vi "dds_host_denzal-final.vi"() -> ()   [LabVIEW 2018]
uses:
  <vilib>/FPGAPlugInAG/PCIe-7841R/niLvFpga_Open_PCIe-7841R.vi
  <vilib>/rvi/interface/common/dynamic/niFpgaDynamicAddResources.vi
  <vilib>/FPGAPlugInAG/Dynamic/niLvFpga_Run_Dynamic.vi
  <vilib>/Utility/error.llb/Error Cluster From Error Code.vi
  <vilib>/rvi/errors/niLvFpgaAdjustHostInterfaceError.vi
  <vilib>/FPGAPlugInAG/Dynamic/niLvFpga_Close_Dynamic.vi
  <vilib>/rvi/interface/nirviOpenFPGA/nirviOpenFPGA.xnode
  FPGA Bitfiles/dds_FPGATarget_ddsfpga_kTR-VUpZgFc _denzal-final.lvbitx
  <vilib>/rvi/interface/nirviMethod/nirviMethod.xnode
  <vilib>/rvi/interface/nirviReadWriteControl/nirviReadWriteControl.xnode
  <vilib>/rvi/interface/nirviCloseFPGA/nirviCloseFPGA.xnode
  <vilib>/rvi/interface/Simulation/niFpgaSimulationCallBeginRW.vi
  NiFpgaLv.dll
  <vilib>/rvi/Analysis/host/Public/NI_FpgaMspHost.lvlib
panel:
  in  "set xz drive":bool
  in  "set yz drive":bool
  out "phi_dc_offset 2":fxp<+/-,17,9>
  out "Actual loop rate 2":u32
  out "Actual Sample Rate (S/s) 2":dbl=952380.9523809524 format="%#_6p"
  in  "change_phi_offset":bool
  in  "filter":bool
  in  "RMS":u16
  in  "noise_scale":fxp<+/-,16,1>
  in  "noise":bool
  out "sine_gen":dbl(graph)
  out "In Range?":bool
  in  "reset_accum":bool
  in  "frequency":u32=100
  in  "sine_amp":dbl=10.0 format="%#_13g"
  in  "xy_amplitude_mod?":bool
  in  "subtract_cross_pol_phi_mean":bool
  in  "phi_fb_out_scale":dbl
  in  "change_phi_dg":bool
  in  "phi_pg":fxp<+/-,16,12>
  in  "change_pm_freq":bool
  in  "phi_dc_offset":fxp<+/-,16,8>
  in  "test_phase_mod":bool
  in  "inst_freq_offset":fxp<+/-,33,18>
  in  "phi_lower_lim":fxp<+/-,16,16>=-1.0
  in  "phi_upper_lim":fxp<+/-,16,16>=1.0
  in  "phi_dg":dbl
  out "phi_fb_out":dbl(graph)
  out "inst_freq":dbl(graph)=22820.240234375
  in  "phi_bitshift":i16
  in  "initialize_phase_mod":bool
  in  "phase_mod":bool
  in  "phase_mod_scale":dbl
  out "phase_out":dbl(graph)=22820.240234375
  in  "phase_mod_param":T1={"Sine wave frequency (Hz)"=50.0, "Phase offset (deg)"=0.0} {"Phase offset (deg)" format="%#_6p"; "Sine wave frequency (Hz)" format="%#_6p"}
  in  "downsample_num":i16=1
  out "cross_pol_phi":dbl(graph)=22820.240234375
  out "actual_analog_in_loop_time":u32=4
  in  "desired_AI_loop_time(uSec)":u32=5
  in  "reset_phi":bool
  in  "discont_pos":fxp<+/-,17,3>=1.0
  in  "discont_neg":fxp<+/-,64,32>=-1.0
  in  "counter_offset":u8
  out "cross_pol_amp":i16(graph)=1
  in  "subtract_mean?":bool=TRUE
  out "slow_freq":dbl=50.0
  out "scale factor_slow-dds":fxp<+/-,16,1>
  in  "vpp_slow-dds":dbl
  in  "slow-dds_param":T1={"Sine wave frequency (Hz)"=50.0, "Phase offset (deg)"=0.0} {"Phase offset (deg)" format="%#_6p"; "Sine wave frequency (Hz)" format="%#_6p"}
  in  "z_slow-dds?":bool
  in  "45_sin":bool=TRUE
  in  "23_sin":bool
  in  "01_sin":bool=TRUE
  in  "just x?":bool
  out "synth_settings_client":dbl[](array[numeric])=[8.0, 50000.0]
  out "scale factor 45":fxp<+/-,16,1>
  out "scale factor 23":fxp<+/-,16,1>
  out "scale factor 01":fxp<+/-,16,1>
  in  "set xy drive":bool
  in  "vpp 45":dbl
  in  "vpp 23":dbl
  in  "vpp 01":dbl
  in  "Desired loop rate (ticks)":u32=88
  in  "frequency increment":dbl=1.0
  out "requested_freq":dbl(graph)=4000.0
  out "Sampling Rate\nAchieved?":bool=TRUE
  out "Actual Sample Rate (S/s)":dbl=952380.9523809524 format="%#_6p"
  in  "re-initialize_dds":bool
  in  "fast-dds_param":T1={"Sine wave frequency (Hz)"=4000.0, "Phase offset (deg)"=0.0} {"Phase offset (deg)" format="%#_6p"; "Sine wave frequency (Hz)" format="%#_6p"}
  in  "step_time (ms)":u32=1
  out "error out":errorcluster={"status"=FALSE, "code"=61003, "source"="niLvFpga_Run_Dynamic.vi"}
  in  "stop":bool
  # "SINE"
  # "COSINE"
  # "SINE"
types:
  T1 = cluster{"Sine wave frequency (Hz)":dbl, "Phase offset (deg)":dbl}
  T2 = enum16{"open", "replace", "create", "open or create", "replace or create", "replace or create with confirmation"}
  T3 = cluster{"frequency (periods/tick)":fxp<+,32,0>, "phase offset (periods)":fxp<+,32,0>, fxp<+/-,16,1>, fxp<+,1,1>}
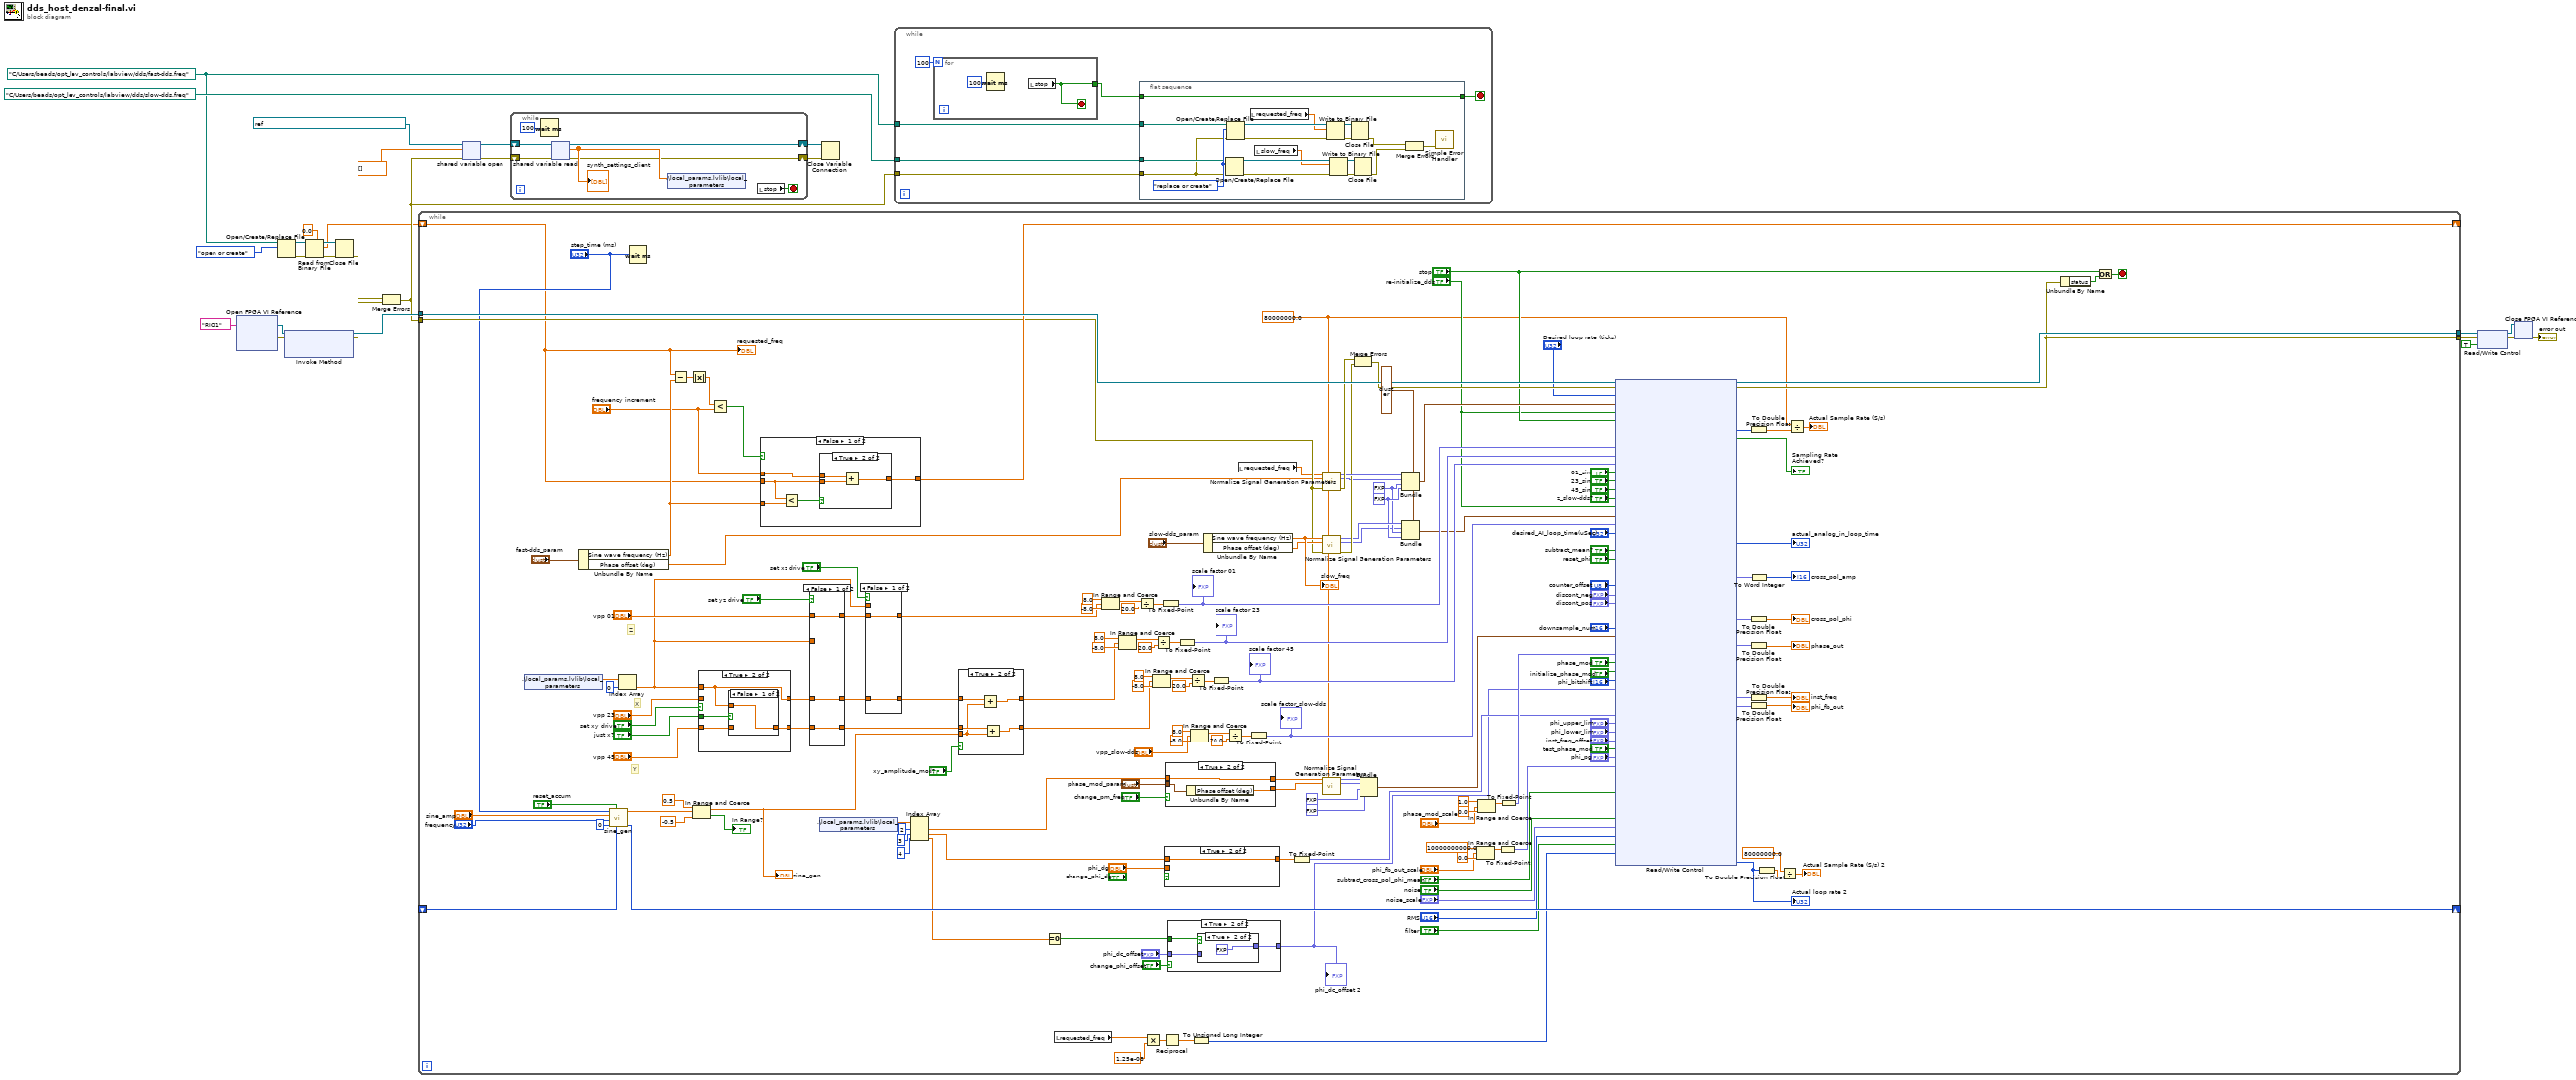
[diagram p0: block diagram]
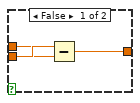
[diagram p8: hidden frame]
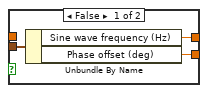
[diagram p10: hidden frame]
diagram:
  w11 = path "C:/Users/beads/opt_lev_controls/labview/dds/fast-dds.freq" ("file path (use dialog)")
  n1 = xnode "Open FPGA VI Reference"("resource name"=tag "RIO1") -> ("FPGA VI Reference Out"=w26:refnum<k20>, "error out"=w27:errorcluster)  [unwired: 1 in]
  n2 = Open/Create/Replace File(file path (use dialog)=w11, operation (0:open)=T2."open or create") -> (refnum out=w9:refnum<file>, error out=w10:errorcluster)  [unwired: 4 in, 1 out]
  n3 = xnode "Invoke Method"("FPGA VI Reference In"=w26, "error in"=w27) -> ("FPGA VI Reference Out"=w25:refnum<k20>, "error out"=w6:errorcluster)  [unwired: 1 in]
  n4 = Read from Binary File(5:0.0, 8:w10, 11:w9) -> (0:w8:errorcluster, 2:w1:dbl, 3:w7:refnum<file>)  [unwired: 3 in, 1 out]
  n5 = Close File(refnum=w7, error in=w8) -> (error out=w5:errorcluster)  [unwired: 1 out]
  n6 = Merge Errors(w5, w6) -> (w2:errorcluster)
  n7 = while {
    tunnel: w25 -> [w202]
    tunnel: w2 -> [w155]
    tunnel: [w200] -> w24
    tunnel: [w201] -> w23
    shift-right: [w180] -> _
    shift-left: w1 -> [w46]
    shift-right: [w67] -> _
    shift-left: _ -> [w66]
    stop <- w198 stop-if-true
    w150 = fxp<+/-,16,1> 0.0
    w153 = T3 {"frequency (periods/tick)"=0.0, "phase offset (periods)"=0.0, 0.0, 0.0} ("cluster")
    w151 = fxp<+,1,1> 0.0
    w121 = 80000000.0 ("FPGA clock rate (Hz)")
    # "Y"
    # "X"
    # "Z"
    n8 = shared-variable ".\\local_params.lvlib\\local_parameters"() -> (w179:dbl[])  [unwired: 1 in, 1 out]
    n9 = Unbundle By Name("fast-dds_param") -> ("Sine wave frequency (Hz)"=w184:dbl, "Phase offset (deg)"=w127:dbl)
    n10 = call "sine_gen.vi"("prev_val"=w66, "reset_accum"="reset_accum", "phase_shift 2"=u32 0, "frequency"="frequency", "sine_amp"="sine_amp", "step_time(ms)"="step_time (ms)") -> ("next_val"=w67:u32, "sine_out"=w61:dbl)  [unwired: 3 in]
    n11 = Index Array(array=w179, index=0) -> (element=w36:dbl)
    n12 = Wait (ms)(milliseconds to wait="step_time (ms)") -> ()  [unwired: 1 out]
    n13 = Subtract(x=w46, y=w184) -> (x-y=w95:dbl)
    n14 = Absolute Value(x=w95) -> (abs(x)=w94:dbl)
    n15 = In Range and Coerce(upper limit=0.5, x=w61, lower limit=-0.5) -> (coerced(x)=w62:dbl, In Range?=→"In Range?":bool)
    "sine_gen" <- w62
    n16 = case shown="True" "set xy drive" {
      tunnel: "vpp 23" -> [w245 _]
      tunnel: [w245 w246] -> w39
      tunnel: "vpp 45" -> [w244 w248]
      tunnel: [w244 w247] -> w38
      tunnel: "just x?" -> [_ w249]
      tunnel: w36 -> [_ w246]
      frame False {
      }
      frame True {
        n17 = case shown="False" w249 {
          tunnel: w248 -> [_ w251]
          tunnel: [w250 w251] -> w247
          tunnel: w246 -> [w250 _]
          frame False {
          }
          frame True {
          }
        }
      }
    }
    n18 = Less?(x=w94, y="frequency increment") -> (x < y?=w92:bool)
    n19 = case shown="False" w92 {
      tunnel: [w227 w237] -> w180
      tunnel: w46 -> [w226 _]
      tunnel: w184 -> [w230 w237]
      tunnel: "frequency increment" -> [w228 _]
      frame False {
        n20 = Less?(x=w226, y=w230) -> (x < y?=w229:bool)
        n21 = case shown="True" w229 {
          tunnel: w226 -> [w232 w236]
          tunnel: w228 -> [w231 w235]
          tunnel: [w233 w234] -> w227
          frame False {
            n22 = Subtract(x=w232, y=w231) -> (x-y=w233:dbl)
          }
          frame True {
            n23 = Add(x=w235, y=w236) -> (x+y=w234:dbl)
          }
        }
      }
      frame True {
      }
    }
    n24 = case shown="False" "set yz drive" {
      tunnel: [w208 w210] -> w35
      tunnel: "vpp 01" -> [w208 _]
      tunnel: w36 -> [_ w210]
      tunnel: [w207 w209] -> w32
      tunnel: w39 -> [w207 w209]
      tunnel: [w206 w210] -> w31
      tunnel: w38 -> [w206 _]
      frame False {
      }
      frame True {
      }
    }
    n25 = shared-variable ".\\local_params.lvlib\\local_parameters"() -> (w99:dbl[])  [unwired: 1 in, 1 out]
    n26 = case shown="False" "set xz drive" {
      tunnel: w36 -> [_ w205]
      tunnel: w35 -> [w204 _]
      tunnel: [w204 w205] -> w34
      tunnel: [w203 w205] -> w33
      tunnel: w32 -> [w203 _]
      frame False {
      }
      frame True {
      }
    }
    n27 = Index Array(array=w99, index #1=2 ("index"), index #2=3 ("index"), index #3=4 ("index")) -> (element #1=w97:dbl, element #2=w89:dbl, element #3=w42:dbl)
    n28 = case shown="True" "xy_amplitude_mod?" {
      tunnel: w33 -> [w218 w223]
      tunnel: [w218 w221] -> w75
      tunnel: w31 -> [w217 w222]
      tunnel: [w217 w220] -> w74
      tunnel: w62 -> [_ w219]
      frame False {
      }
      frame True {
        n29 = Add(x=w223, y=w219) -> (x+y=w221:dbl)
        n30 = Add(x=w222, y=w219) -> (x+y=w220:dbl)
      }
    }
    n31 = Equal To 0?(x=w42) -> (x = 0?=w53:bool)
    n32 = local read "requested_freq"() -> (w29:dbl)
    n33 = In Range and Coerce(upper limit=8.0, x=w34, lower limit=-8.0) -> (coerced(x)=w187:dbl)  [unwired: 1 out]
    n34 = In Range and Coerce(upper limit=8.0, x=w75, lower limit=-8.0) -> (coerced(x)=w168:dbl)  [unwired: 1 out]
    n35 = Divide(x=w187, y=20.0) -> (x/y=w193:dbl)
    n36 = Multiply(x=w29, y=1.25e-08) -> (x*y=w45:dbl)
    n37 = In Range and Coerce(upper limit=8.0, x=w74, lower limit=-8.0) -> (coerced(x)=w162:dbl)  [unwired: 1 out]
    n38 = Divide(x=w168, y=20.0) -> (x/y=w169:dbl)
    n39 = To Fixed-Point(number=w193) -> (fixed-point=w182:fxp<+/-,16,1>)  [unwired: 1 in]
    "scale factor 01" <- w182
    n40 = Reciprocal(x=w45) -> (1/x=w44:dbl)
    n41 = case shown="True" "change_phi_dg" {
      tunnel: w89 -> [_ w225]
      tunnel: [w224 w225] -> w88
      tunnel: "phi_dg" -> [w224 _]
      frame False {
      }
      frame True {
      }
    }
    n42 = case shown="True" "change_pm_freq" {
      tunnel: "phase_mod_param" -> [w240 w243]
      tunnel: [w239 w242] -> w123
      tunnel: [w238 w241] -> w122
      tunnel: w97 -> [_ w242]
      frame False {
        n43 = Unbundle By Name(w240) -> ("Sine wave frequency (Hz)"=w239:dbl, "Phase offset (deg)"=w238:dbl)
      }
      frame True {
        n44 = Unbundle By Name(w243) -> ("Phase offset (deg)"=w241:dbl)
      }
    }
    n45 = case shown="True" "change_phi_offset" {
      tunnel: [w211 w213] -> w55
      tunnel: "phi_dc_offset" -> [w211 w212]
      tunnel: w53 -> [_ w214]
      frame False {
      }
      frame True {
        n46 = case shown="True" w214 {
          tunnel: [w215 fxp<+/-,16,8> 0.0] -> w213
          tunnel: w212 -> [w215 _]
          frame False {
          }
          frame True {
          }
        }
      }
    }
    "phi_dc_offset 2" <- w55
    n47 = To Fixed-Point(number=w169) -> (fixed-point=w165:fxp<+/-,16,1>)  [unwired: 1 in]
    "scale factor 23" <- w165
    n48 = Divide(x=w162, y=20.0) -> (x/y=w163:dbl)
    n49 = In Range and Coerce(upper limit=8.0, x="vpp_slow-dds", lower limit=-8.0) -> (coerced(x)=w146:dbl)  [unwired: 1 out]
    n50 = To Unsigned Long Integer(number=w44) -> (unsigned 32bit integer=w48:u32)
    n51 = Unbundle By Name("slow-dds_param") -> ("Sine wave frequency (Hz)"=w157:dbl, "Phase offset (deg)"=w156:dbl)
    "slow_freq" <- w157
    n52 = To Fixed-Point(number=w163) -> (fixed-point=w159:fxp<+/-,16,1>)  [unwired: 1 in]
    "scale factor 45" <- w159
    n53 = Divide(x=w146, y=20.0) -> (x/y=w147:dbl)
    n54 = local read "requested_freq"() -> (w30:dbl)
    n55 = To Fixed-Point(number=w147) -> (fixed-point=w142:fxp<+/-,16,1>)  [unwired: 1 in]
    "scale factor_slow-dds" <- w142
    n56 = To Fixed-Point(number=w88) -> (fixed-point=w85:fxp<+/-,32,16>)  [unwired: 1 in]
    n57 = call <vilib>:"Normalize Signal Generation Parameters.vi"("frequency (Hz)"=w30, "FPGA clock rate (Hz)"=w121, "phase offset (deg)"=w127, "error in (no error)"=w155) -> ("frequency (periods/tick)"=w195:fxp<+,32,0>, "phase offset (periods)"=w125:fxp<+,32,0>, "error out"=w197:errorcluster)  [unwired: 6 in, 3 out]
    n58 = call <vilib>:"Normalize Signal Generation Parameters.vi"("frequency (Hz)"=w157, "FPGA clock rate (Hz)"=w121, "phase offset (deg)"=w156, "error in (no error)"=w155) -> ("frequency (periods/tick)"=w152:fxp<+,32,0>, "phase offset (periods)"=w126:fxp<+,32,0>, "error out"=w154:errorcluster)  [unwired: 6 in, 3 out]
    n59 = call <vilib>:"Normalize Signal Generation Parameters.vi"("frequency (Hz)"=w123, "FPGA clock rate (Hz)"=w121, "phase offset (deg)"=w122) -> ("frequency (periods/tick)"=w120:fxp<+,32,0>, "phase offset (periods)"=w119:fxp<+,32,0>)  [unwired: 7 in, 4 out]
    n60 = Merge Errors(w197, w154) -> (w196:errorcluster)
    n61 = Bundle("frequency (periods/tick)"=w120, "phase offset (periods)"=w119, fxp<+/-,16,1> 0.0, fxp<+,1,1> 0.0) -> (w118:T3)  [unwired: 1 in]
    n62 = Bundle(cluster=w153, "frequency (periods/tick)"=w195, "phase offset (periods)"=w125, w150, w151) -> (w192:T3)
    n63 = Bundle(cluster=w153, "frequency (periods/tick)"=w152, "phase offset (periods)"=w126, w150, w151) -> (w149:T3)
    n64 = In Range and Coerce(upper limit=10000000000.0, x="phi_fb_out_scale", lower limit=0.0) -> (coerced(x)=w81:dbl)  [unwired: 1 out]
    n65 = In Range and Coerce(upper limit=1.0, x="phase_mod_scale", lower limit=0.0) -> (coerced(x)=w111:dbl)  [unwired: 1 out]
    n66 = To Fixed-Point(number=w81) -> (fixed-point=w80:fxp<+/-,16,16>)  [unwired: 1 in]
    n67 = To Fixed-Point(number=w111) -> (fixed-point=w91:fxp<+,16,0>)  [unwired: 1 in]
    n68 = xnode "Read/Write Control"("FPGA VI Reference In"=w202, "error in"=w196, "Desired loop rate (ticks)"="Desired loop rate (ticks)", "sinewave-props_fast-dds"=w192, "Initialize fast-dds"="re-initialize_dds", "stop"="stop", "fast-dds_scale01"=w182, "fast-dds_scale23"=w165, "fast-dds_scale45"=w159, "01_sin"="01_sin", "23_sin"="23_sin", "45_sin"="45_sin", "z_slow-dds?"="z_slow-dds?", "Initialize slow-dds"="re-initialize_dds", "sinewave-props_slow-dds"=w149, "slow-dds_scale"=w142, "desired_analog_in_loop_time_(uSec)"="desired_AI_loop_time(uSec)", "subtract_mean"="subtract_mean?", "reset_phi"="reset_phi", "counter_offset"="counter_offset", "discont_neg"="discont_neg", "discont_pos"="discont_pos", "downsample_num"="downsample_num", "phase_mod_props"=w118, "phase_mod_scale"=w91, "phase_mod"="phase_mod", "initialize_phase_mod"="initialize_phase_mod", "phi_bitshift"="phi_bitshift", "phi_dc_offset"=w55, "phi_dg"=w85, "phi_upper_lim"="phi_upper_lim", "phi_lower_lim"="phi_lower_lim", "inst_freq_offset"="inst_freq_offset", "test_phase_mod"="test_phase_mod", "phi_pg"="phi_pg", "phi_fb_out_scale"=w80, "subtract_cross_pol_phi_mean"="subtract_cross_pol_phi_mean", "noise"="noise", "noise_scale"="noise_scale", "RMS"="RMS", "filter"="filter", "Desired loop rate (ticks) 2"=w48) -> ("FPGA VI Reference Out"=w201:refnum<k20>, "error out"=w200:errorcluster, "Actual loop rate"=w189:u32, "Sampling rate achieved?"=→"Sampling Rate\nAchieved?":bool, "actual_analog_in_loop_time"=→"actual_analog_in_loop_time":u32, "cross_pol_amp"=w140:fxp<+,32,16>, "phi_full_out"=w131:fxp<+/-,35,21>, "phase_mod_out"=w115:fxp<+/-,49,17>, "inst_freq"=w107:fxp<+/-,35,20>, "phi_fb_out"=w104:fxp<+/-,32,0>, "Actual loop rate 2"=w50:u32)  [unwired: 1 in, 5 out]
    "Actual loop rate 2" <- w50
    n69 = To Double Precision Float(number=w189) -> (double precision float=w191:dbl)
    n70 = To Word Integer(number=w140) -> (16bit integer=→"cross_pol_amp":i16)
    n71 = To Double Precision Float(number=w131) -> (double precision float=→"cross_pol_phi":dbl)
    n72 = To Double Precision Float(number=w115) -> (double precision float=→"phase_out":dbl)
    n73 = To Double Precision Float(number=w107) -> (double precision float=→"inst_freq":dbl)
    n74 = To Double Precision Float(number=w104) -> (double precision float=→"phi_fb_out":dbl)
    n75 = To Double Precision Float(number=w50) -> (double precision float=w52:dbl)
    n76 = Divide(x=80000000.0, y=w52) -> (x/y=→"Actual Sample Rate (S/s) 2":dbl)
    n77 = Divide(x=w121, y=w191) -> (x/y=→"Actual Sample Rate (S/s)":dbl)
    n78 = Unbundle By Name(w200) -> ("status"=w199:bool)
    n79 = Or(x="stop", y=w199) -> (x .or. y?=w198:bool)
    "requested_freq" <- w46
  }
  n80 = shared-variable-open(refnum<k21> "ni.var.psp://localhost/daq_lib/synth_settings" ("shared variable refnum in"), w2, dbl[] [] ("synth_settings_client")) -> (w16:refnum<k21>, w15:errorcluster)  [unwired: 1 in]
  n81 = while {
    shift-right: [w253] -> w14
    shift-left: w16 -> [w256]
    shift-right: [w252] -> w13
    shift-left: w15 -> [w255]
    stop <- w257 stop-if-true
    n82 = Wait (ms)(milliseconds to wait=u32 100) -> ()  [unwired: 1 out]
    n83 = shared-variable-read(w256, w255) -> (w253:refnum<k21>, w252:errorcluster, w254:dbl[])  [unwired: 1 out]
    "synth_settings_client" <- w254
    n84 = shared-variable ".\\local_params.lvlib\\local_parameters"(w254) -> ()  [unwired: 1 in, 1 out]
    n85 = local read "stop"() -> (w257:bool)
  }
  n86 = Close Variable Connection(8:w13, 11:w14) -> ()  [unwired: 1 out]
  n87 = while {
    tunnel: w11 -> [w264]
    tunnel: path "C:/Users/beads/opt_lev_controls/labview/dds/slow-dds.freq" ("file path (use dialog)") -> [w263]
    tunnel: w2 -> [w261]
    stop <- w259 stop-if-true
    n88 = for {
      N: 100 -> [_]
      tunnel: [w284] -> w260
      stop <- w284 stop-if-true
      n89 = Wait (ms)(milliseconds to wait=u32 100) -> ()  [unwired: 1 out]
      n90 = local read "stop"() -> (w284:bool)
    }
    n91 = flat-sequence {
      tunnel: w264 -> [w268]
      tunnel: w263 -> [w267]
      tunnel: w261 -> [w266]
      tunnel: w260 -> [w265]
      tunnel: [w265] -> w259
      frame #0 {
        w282 = T2."replace or create" ("operation (0:open)")
        n92 = Open/Create/Replace File(file path (use dialog)=w267, error in=w266, operation (0:open)=w282) -> (refnum out=w277:refnum<file>, error out=w278:errorcluster)  [unwired: 3 in, 1 out]
        n93 = Open/Create/Replace File(file path (use dialog)=w268, error in=w266, operation (0:open)=w282) -> (refnum out=w281:refnum<file>, error out=w280:errorcluster)  [unwired: 3 in, 1 out]
        n94 = local read "requested_freq"() -> (w279:dbl)
        n95 = local read "slow_freq"() -> (w276:dbl)
        n96 = Write to Binary File(file (use dialog)=w281, data=w279, error in=w280) -> (refnum out=w274:refnum<file>, error out=w275:errorcluster)  [unwired: 3 in, 1 out]
        n97 = Write to Binary File(file (use dialog)=w277, data=w276, error in=w278) -> (refnum out=w273:refnum<file>, error out=w272:errorcluster)  [unwired: 3 in, 1 out]
        n98 = Close File(refnum=w274, error in=w275) -> (error out=w271:errorcluster)  [unwired: 1 out]
        n99 = Close File(refnum=w273, error in=w272) -> (error out=w270:errorcluster)  [unwired: 1 out]
        n100 = Merge Errors(w271, w270) -> (w269:errorcluster)
        n101 = call <vilib>:"Simple Error Handler.vi"("error in (no error)"=w269) -> ()  [unwired: 4 in, 5 out]
      }
    }
  }
  n102 = xnode "Read/Write Control"("FPGA VI Reference In"=w23, "error in"=w24, "stop"=TRUE) -> ("FPGA VI Reference Out"=w22:refnum<k20>, "error out"=w21:errorcluster)
  n103 = xnode "Close FPGA VI Reference"("FPGA VI Reference In"=w22, "error in"=w21) -> ("error out"=→"error out":errorcluster)
